vi "ForceSettings.vi"(9 "Function":i32) -> (1 "k":dbl format="%#_13g", 2 "Setpoint":dbl format="%#_13g")   [LabVIEW 2023]
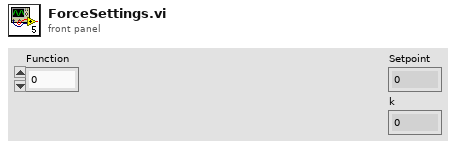
[diagram p1: front panel]
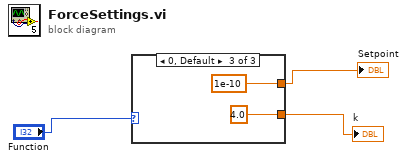
[diagram p0: block diagram]
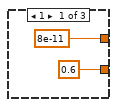
[diagram p2: hidden frame]
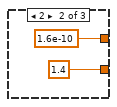
[diagram p3: hidden frame]
diagram:
  n1 = case shown="0, Default" "Function" {
    tunnel: [0.6 1.4 4.0] -> w3
    tunnel: [8e-11 1.6e-10 1e-10] -> w2
    frame 1 {
    }
    frame 2 {
    }
    frame 0, Default {
    }
  }
  "Setpoint" <- w2
  "k" <- w3
